vi "Filename Incrementer.vi"(11 "File Path":path) -> (3 "File Path out":path)   [LabVIEW 2017, in "Test Executive Builder Model.lvclass"]
uses:
  <vilib>/gpm_packages/@cs/Test-executive-builder/Source/Test Executive Builder Model/Test Executive Builder Model/Test Executive Builder Model.lvclass
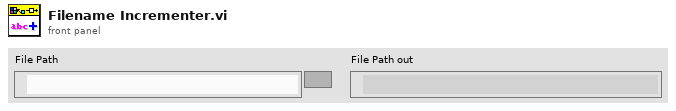
[diagram p1: front panel]
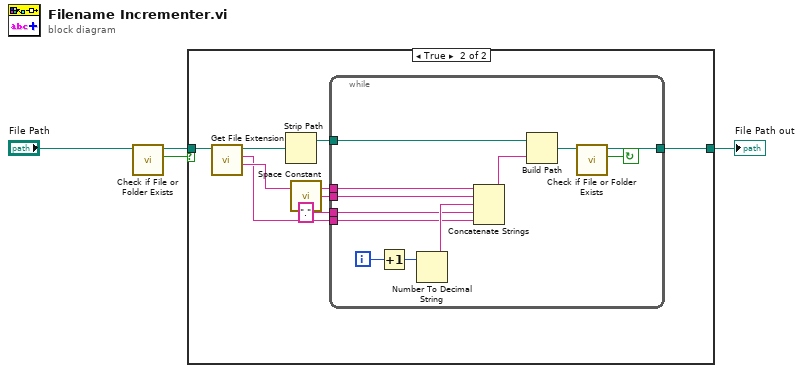
[diagram p0: block diagram]
diagram:
  n1 = call <vilib>:"Check if File or Folder Exists.vi"("path"="File Path") -> ("file or folder exists?"=w3:bool, "dup path"=w2:path)  [unwired: 8 in, 1 out]
  n2 = case shown="True" w3 {
    tunnel: w2 -> [w5 w12]
    tunnel: [w5 w7] -> w1
    frame False {
    }
    frame True {
      n3 = call <vilib>:"Get File Extension.vi"("file"=w12) -> ("filename without extension"=w10:string, "lowercase file extension"=w9:string, "dup file"=w11:path)  [unwired: 6 in, 2 out]
      n4 = Strip Path(path=w11) -> (stripped path=w13:path)  [unwired: 1 out]
      n5 = call <vilib>:"Space Constant.vi"() -> ("String"=w8:string)
      n6 = while {
        tunnel: w13 -> [w20]
        tunnel: w10 -> [w25]
        tunnel: w9 -> [w15]
        tunnel: w8 -> [w24]
        tunnel: [w16] -> w7
        tunnel: "." ("string") -> [w14]
        i -> [w23]
        stop <- w17 continue-if-true
        n7 = Increment(x=w23) -> (x+1=w22:i32)
        n8 = Number To Decimal String(number=w22) -> (decimal integer string=w21:string)  [unwired: 1 in]
        n9 = Concatenate Strings(w25, w24, w21, w14, w15) -> (w19:string)
        n10 = Build Path(base path=w20, name or relative path=w19) -> (appended path=w18:path)
        n11 = call <vilib>:"Check if File or Folder Exists.vi"("path"=w18) -> ("file or folder exists?"=w17:bool, "dup path"=w16:path)  [unwired: 8 in, 1 out]
      }
    }
  }
  "File Path out" <- w1
